vi "Write LHW-Data Objects.vi"(8 "error in (no error)":errorcluster, 10 "LHW-Data Objects":refnum<class "LHW-Data.lvclass">[](array[class]), 11 "LHW-DataCollection in":refnum<class "LHW-DataCollection.lvclass">) -> (0 "error out":errorcluster, 3 "LHW-DataCollection out":refnum<class "LHW-DataCollection.lvclass">)   [LabVIEW 2014, in "LHW-Data.lvlib" / "LHW-DataCollection.lvclass"]
doc: "Write LHW-DataObjects to Attribute."
uses:
  LHW-DataCollection.lvclass
  LHW-Data/LHW-Data.lvclass
  LHW-DataCollection.lvclass/LHW-DataCollection.ctl
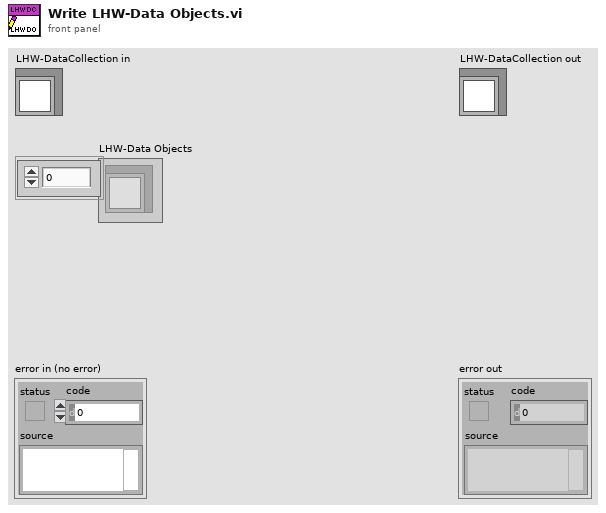
[diagram p1: front panel]
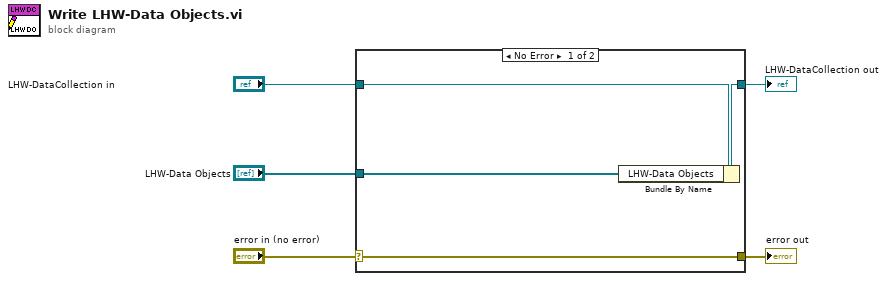
[diagram p0: block diagram]
diagram:
  n1 = case shown="No Error" "error in (no error)" {
    selector: "error in (no error)" -> [w9 w10]
    tunnel: [w9 w10] -> w4
    tunnel: [w7 w11] -> w2
    tunnel: "LHW-DataCollection in" -> [w8 w11]
    tunnel: "LHW-Data Objects" -> [w6 _]
    frame No Error {
      n2 = Bundle By Name(cluster=w8, "LHW-Data Objects"=w6) -> (w7:refnum<class "LHW-DataCollection.lvclass">)
    }
    frame Error {
    }
  }
  "error out" <- w4
  "LHW-DataCollection out" <- w2
